vi "Test - Using Traverse.vi"   [LabVIEW 2019]
doc: "This test VI is used by the Using Traverse.vi example."
uses:
  <vilib>/Utility/file.llb/Write Delimited Spreadsheet (DBL).vi
panel:
  # "DO NOT SAVE CHANGES TO THIS VI. This VI serves as the target for the Using Traverse.vi example. Therefore, changing this VI might prevent the Using Traverse.vi example from demonstrating its scripting task."
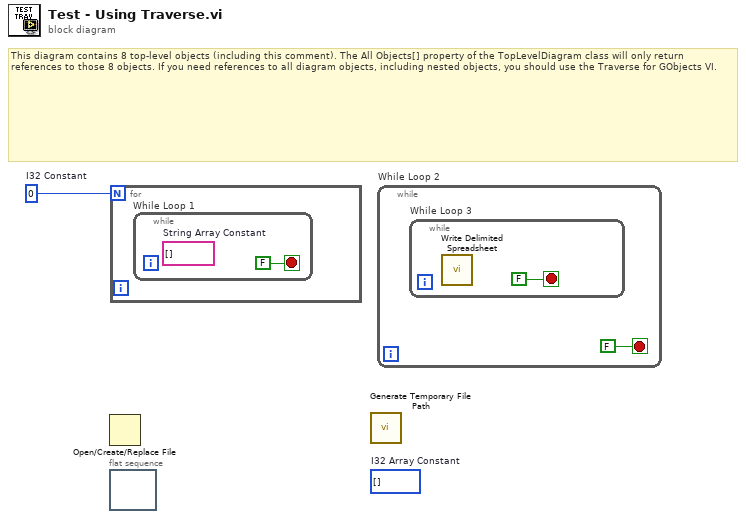
[diagram p0: block diagram]
diagram:
  w1 = 0  # I32 Constant
  (unwired) i32[] []  # I32 Array Constant
  # "This diagram contains 8 top-level objects (including this comment). The All Objects[] property of the TopLevelDiagram class will only return references to those 8 objects. If you need references to all diagram objects, including nested objects, you should use the Traverse for GObjects VI."
  n1 = Open/Create/Replace File() -> ()  [unwired: 6 in, 3 out]
  n2 = flat-sequence {
    frame #0 {
    }
  }
  n3 = for {
    N: w1 -> [_]
    n4 = while "While Loop 1" {
      stop <- FALSE stop-if-true
      (unwired) string[] []  # String Array Constant
    }
  }
  n5 = call <vilib>:"Generate Temporary File Path.vi"() -> ()  [unwired: 10 in, 2 out]
  n6 = while "While Loop 2" {
    stop <- FALSE stop-if-true
    n7 = while "While Loop 3" {
      stop <- FALSE stop-if-true
      n8 = call-poly <vilib>:"Write Delimited Spreadsheet.vi"() -> ()  [unwired: 14 in, 2 out]
    }
  }
